vi "onUnsubscribe.vi"(6 "timeout (100ms)":i32=100, 8 "error in (no error)":errorcluster, 10 "UNSUBSCRIBE":refnum<class "UNSUBSCRIBE.lvclass">, 11 "Client in":refnum<class "Client.lvclass">) -> (0 "error out":errorcluster, 2 "UNSUBACK":refnum<class "UNSUBACK.lvclass">, 3 "Client out":refnum<class "Client.lvclass">)   [LabVIEW 2013, in "MQTT Client.lvlib" / "Client.lvclass"]
uses:
  Client.lvclass
  <vilib>/LabVIEW Open Source Project/MQTT Control Packets/Control Packets/UNSUBSCRIBE/UNSUBSCRIBE.lvclass
  <vilib>/LabVIEW Open Source Project/MQTT Control Packets/Control Packets/UNSUBACK/UNSUBACK.lvclass
  MQTT_Base/Base Class/MQTT_Base.lvclass
  Client.lvclass/Client.ctl
  Session.Client/Session.Client.lvclass
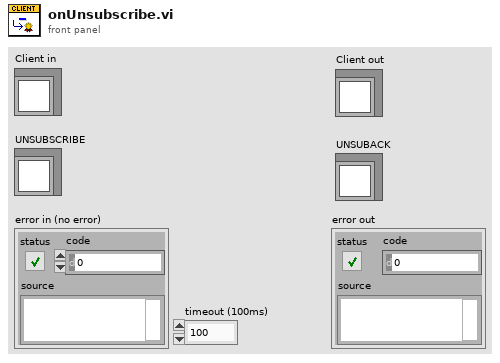
[diagram p1: front panel]
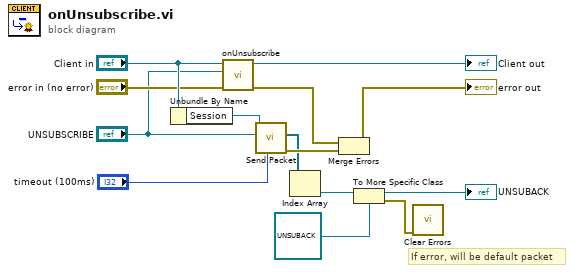
[diagram p0: block diagram]
diagram:
  # "If error, will be default packet"
  n1 = Unbundle By Name("Client in") -> ("Session"=w14:refnum<class "Session.Client.lvclass">)
  n2 = call-parent "onUnsubscribe.vi"("error in (no error)"="error in (no error)", "UNSUBSCRIBE"="UNSUBSCRIBE", "MQTT_Base in"="Client in") -> ("error out"=w12:errorcluster, "MQTT_Base out"=→"Client out":refnum<class "Client.lvclass">)  [unwired: 6 in, 1 out]
  n3 = call "Send Packet.vi"("timeout (0ms : no ack)"="timeout (100ms)", "Packet"="UNSUBSCRIBE", "Session"=w14) -> ("error out"=w13:errorcluster, "Response"=w3:refnum<class "ControlPacket.lvclass">[])  [unwired: 5 in, 2 out]
  n4 = Index Array(array=w3) -> (element=w5:refnum<class "ControlPacket.lvclass">)  [unwired: 1 in]
  n5 = Merge Errors(w12, w13) -> (→"error out":errorcluster)
  n6 = To More Specific Class(target class=refnum<class "UNSUBACK.lvclass"> refnum ("UNSUBACK"), reference=w5) -> (specific class reference=→"UNSUBACK":refnum<class "UNSUBACK.lvclass">, error out=w4:errorcluster)  [unwired: 1 in]
  n7 = call <vilib>:"Clear Errors.vi"("error in (no error)"=w4) -> ()  [unwired: 6 in, 1 out]
